vi "niFpgaBFGroupFirst.vi"(0 "reset":bool, 1 "mult output type":fxp<+/-,18,2> format="%.17g", 2 "bf bullet type":fxp<+/-,16,1> format="%.16g", 5 "bf data in":T1 {"x_r" format="%.16g"; "x_i" format="%.16g"; "y_r" format="%.16g"; "y_i" format="%.16g"}, 7 "stage switch in":bool, 9 "tf index in":fxp<+,10,10>, 11 "bf data type":T1 {"x_r" format="%.16g"; "x_i" format="%.16g"; "y_r" format="%.16g"; "y_i" format="%.16g"}) -> (6 "bf data out":T1 {"x_r" format="%.16g"; "x_i" format="%.16g"; "y_r" format="%.16g"; "y_i" format="%.16g"}, 8 "stage switch out":bool, 10 "tf index out":fxp<+,10,10>)   [LabVIEW 2017]
uses:
  <vilib>/rvi/FXPMathLib/basic elements/FxpDiscreteDelay/XNode/nifxpmath_DiscreteDelay.xnode
  <vilib>/rvi/Analysis/measure/FFT/supportingXNodes/permutation/XNode/niFpgaFFTPermutation.xnode
  <vilib>/rvi/Analysis/measure/FFT/supportingXNodes/butterfly/XNode/niFpgaFFTDIFButterfly.xnode
  <vilib>/rvi/FXPMathLib/FxpMul/XNode/nifxpmath_Multiplier.xnode
  <vilib>/rvi/FXPMathLib/sim/FxpSim.dll
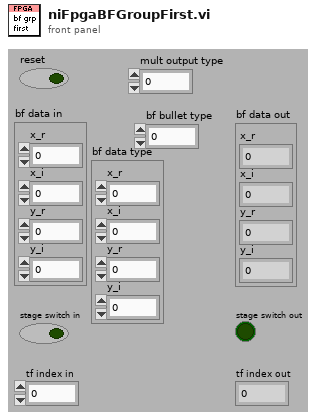
[diagram p1: front panel]
types:
  T1 = cluster{"x_r":fxp<+/-,16,1>, "x_i ":fxp<+/-,16,1>, "y_r ":fxp<+/-,16,1>, "y_i ":fxp<+/-,16,1>}
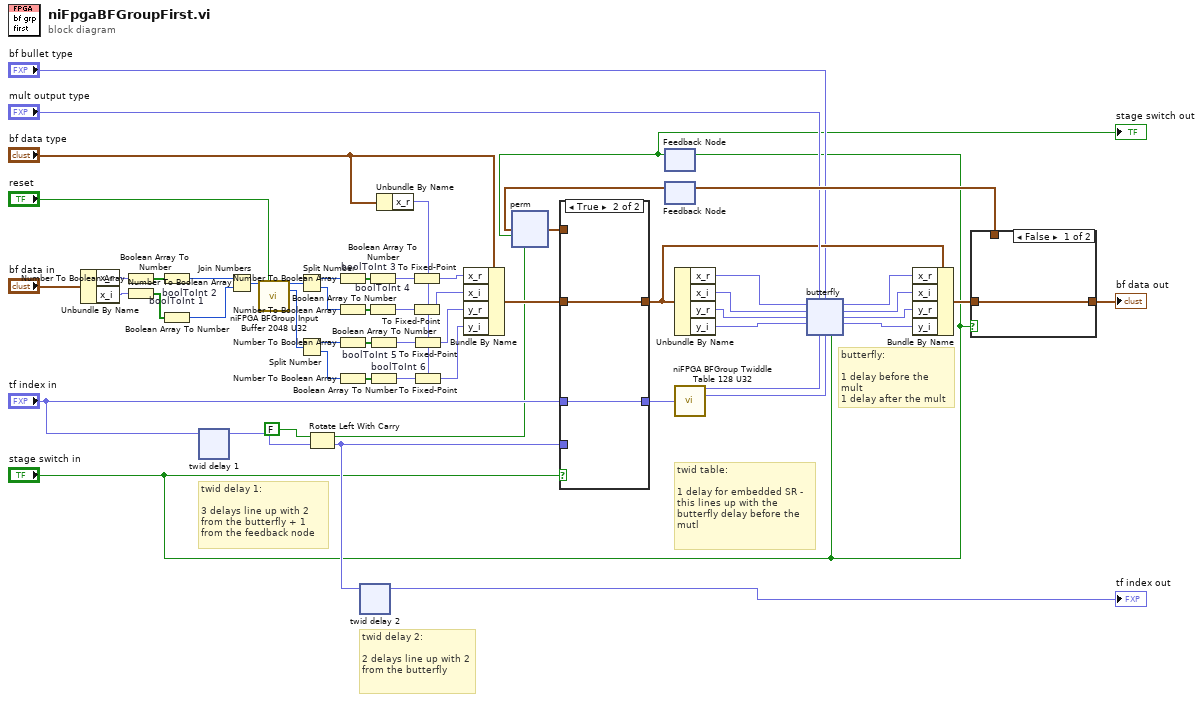
[diagram p0: block diagram]
diagram:
  # "twid delay 2:\n\n2 delays line up with 2 from the butterfly"
  # "twid delay 1:\n\n3 delays line up with 2 from the butterfly + 1 from the feedback node"
  # "twid table:\n\n1 delay for embedded SR - this lines up with the butterfly delay before the mutl"
  # "butterfly: \n\n1 delay before the mult\n1 delay after the mult"
  n1 = Unbundle By Name("bf data in") -> ("x_r"=w23:fxp<+/-,16,1>, "x_i"=w22:fxp<+/-,16,1>)
  n2 = Number To Boolean Array(number=w23) -> (Boolean array=w54:bool[])
  n3 = Number To Boolean Array(number=w22) -> (Boolean array=w53:bool[])
  n4 = Boolean Array To Number "boolToInt 1"(Boolean array=w54) -> (number=w52:u16)
  n5 = Boolean Array To Number "boolToInt 2"(Boolean array=w53) -> (number=w51:u16)
  n6 = xnode "twid delay 1"("D"="tf index in") -> ("Q"=w19:fxp<+,10,10>)
  n7 = Join Numbers(hi=w52, lo=w51) -> ((hi.lo)=w50:u32)
  n8 = call <vilib>:"niFPGA BFGroup Input Buffer 2048 U32.vi"("data in"=w50, "reset"="reset") -> ("x out"=w26:u32, "y out"=w25:u32)  [unwired: 1 in, 11 out]
  n9 = Split Number(x=w26) -> (hi(x)=w48:u16, lo(x)=w45:u16)
  n10 = Split Number(x=w25) -> (hi(x)=w43:u16, lo(x)=w41:u16)
  n11 = Rotate Left With Carry(2:w19, 3:FALSE ("carry")) -> (0:w18:fxp<+,10,10>, 1:w13:bool)
  n12 = Number To Boolean Array(number=w48) -> (Boolean array=w47:bool[])
  n13 = Number To Boolean Array(number=w45) -> (Boolean array=w46:bool[])
  n14 = Number To Boolean Array(number=w43) -> (Boolean array=w44:bool[])
  n15 = Number To Boolean Array(number=w41) -> (Boolean array=w42:bool[])
  n16 = xnode "twid delay 2"("D"=w18) -> ("Q"=→"tf index out":fxp<+,10,10>)
  n17 = Boolean Array To Number "boolToInt 3"(Boolean array=w47) -> (number=w9:fxp<+/-,16,1>)
  n18 = Boolean Array To Number "boolToInt 4"(Boolean array=w46) -> (number=w7:fxp<+/-,16,1>)
  n19 = Boolean Array To Number "boolToInt 5"(Boolean array=w44) -> (number=w5:fxp<+/-,16,1>)
  n20 = Boolean Array To Number "boolToInt 6"(Boolean array=w42) -> (number=w6:fxp<+/-,16,1>)
  n21 = Unbundle By Name("bf data type") -> ("x_r"=w1:fxp<+/-,16,1>)
  n22 = To Fixed-Point(fixed-point type=w1, number=w9) -> (fixed-point=w8:fxp<+/-,16,1>)
  n23 = To Fixed-Point(fixed-point type=w1, number=w7) -> (fixed-point=w2:fxp<+/-,16,1>)
  n24 = To Fixed-Point(fixed-point type=w1, number=w5) -> (fixed-point=w4:fxp<+/-,16,1>)
  n25 = To Fixed-Point(fixed-point type=w1, number=w6) -> (fixed-point=w3:fxp<+/-,16,1>)
  n26 = Bundle By Name(cluster="bf data type", "x_r"=w8, "x_i"=w2, "y_r"=w4, "y_i"=w3) -> (w40:T1)
  n27 = feedback-in #1("stage switch in") -> ()
  n28 = feedback #1() -> (w14:bool)  [unwired: 1 out]
  "stage switch out" <- w14
  n29 = feedback #2() -> (w15:T1)  [unwired: 1 out]
  n30 = xnode "perm"("bf data in"=w15, "stage switch"=w14, "perm switch"=w13) -> ("bf data out"=w16:T1)
  n31 = case shown="True" "stage switch in" {
    tunnel: w16 -> [w58 _]
    tunnel: "tf index in" -> [_ w61]
    tunnel: [w59 w61] -> w39
    tunnel: w18 -> [w59 _]
    tunnel: [w58 w60] -> w27
    tunnel: w40 -> [_ w60]
    frame False {
    }
    frame True {
    }
  }
  n32 = Unbundle By Name(w27) -> ("x_r"=w38:fxp<+/-,16,1>, "x_i"=w37:fxp<+/-,16,1>, "y_r"=w36:fxp<+/-,16,1>, "y_i"=w35:fxp<+/-,16,1>)
  n33 = call <vilib>:"niFPGA BFGroup Twiddle Table 128 U32.vi"("address"=w39) -> ("twid real"=w30:fxp<+/-,17,2>, "twid imag"=w11:fxp<+/-,17,2>)  [unwired: 13 out]
  n34 = xnode "butterfly"("x_r"=w38, "x_i"=w37, "y_r"=w36, "y_i"=w35, "tf_r"=w30, "tf_i"=w11, "mult output type"="mult output type", "bf bullet type"="bf bullet type", "first stage"="stage switch in") -> ("x_out_r"=w34:fxp<+/-,16,1>, "x_out_i"=w33:fxp<+/-,16,1>, "y_out_r"=w32:fxp<+/-,16,1>, "y_out_i"=w31:fxp<+/-,16,1>)
  n35 = Bundle By Name(cluster=w27, "x_r"=w34, "x_i"=w33, "y_r"=w32, "y_i"=w31) -> (w28:T1)
  n36 = case shown="False" "stage switch in" {
    tunnel: [_ w63] -> w55
    tunnel: w28 -> [w62 w63]
    tunnel: [w62 _] -> w56
    frame False {
    }
    frame True {
    }
  }
  "bf data out" <- w56
  n37 = feedback-in #2(w55) -> ()
